vi "start.vi"(8 "error in (no error)":errorcluster, 11 "Model in":refnum<class "Model.lvclass">) -> (0 "error out":errorcluster, 3 "Model out":refnum<class "Model.lvclass">)   [LabVIEW 2013, in "Model.lvclass"]
uses:
  Model.lvclass
  Model.lvclass/Model.ctl
  <userlib>/Common/ILC/ILC/ILC.lvclass
  <userlib>/Common/Devices/FlukeDMM/FlukeDMM/FlukeDMM.lvclass
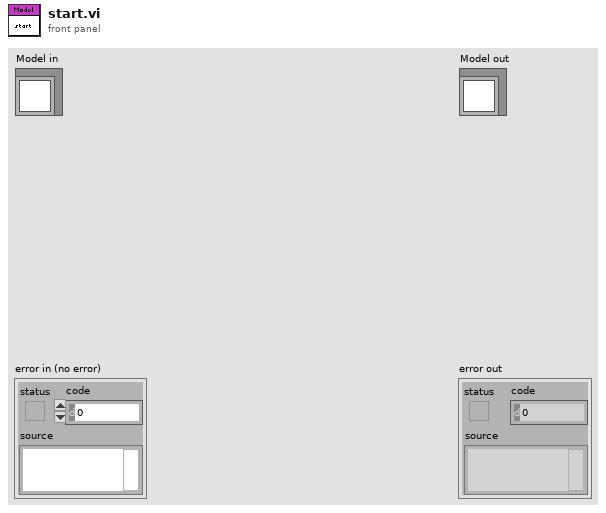
[diagram p1: front panel]
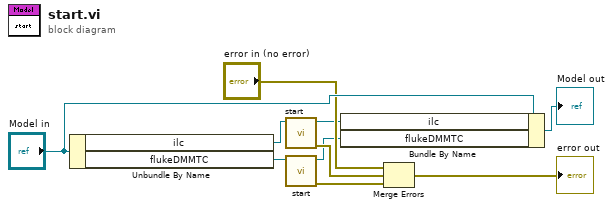
[diagram p0: block diagram]
diagram:
  n1 = Unbundle By Name("Model in") -> ("ilc"=w8:refnum<class "ILC.lvclass">, "flukeDMMTC"=w3:refnum<class "FlukeDMMTC.lvclass">)
  n2 = call <userlib>:"start.vi"("ILC in"=w8) -> ("error out"=w7:errorcluster, "ILC out"=w4:refnum<class "ILC.lvclass">)  [unwired: 9 in]
  n3 = call <userlib>:"start.vi"("FlukeDMM in"=w3) -> ("error out"=w2:errorcluster, "FlukeDMM out"=w1:refnum<class "FlukeDMMTC.lvclass">)  [unwired: 9 in]
  n4 = Bundle By Name(cluster="Model in", "ilc"=w4, "flukeDMMTC"=w1) -> (→"Model out":refnum<class "Model.lvclass">)
  n5 = Merge Errors("error in (no error)", w7, w2) -> (→"error out":errorcluster)
